vi "test-discretization-13.vi"(8 "error in (no error)":errorcluster) -> (0 "error out":errorcluster, 3 "All Tests Passed":bool)   [LabVIEW 2019]
uses:
  <vilib>/Analysis/Matrix/Datatypes/RealMatrix.ctl
  <vilib>/Analysis/_algsub.llb/Matrix Norm Type.ctl
  <vilib>/Analysis/_algsub.llb/Real Matrix Norm.vi
  <vilib>/Rock Robotics/WPI/ThirdParty/JAS_Junk/TrajLib/MatBuilder_Create.vi
  <vilib>/Rock Robotics/WPI/ThirdParty/JAS_Junk/TrajLib/MatrixHelper_CoerceSize.vi
  <vilib>/Rock Robotics/WPI/ThirdParty/JAS_Junk/TrajLib/Matrix_Transpose.vi
  <vilib>/Rock Robotics/WPI/ThirdParty/JAS_Junk/TrajLib/Matrix_AssignBlock.vi
  <vilib>/Rock Robotics/WPI/ThirdParty/JAS_Junk/TrajLib/Matrix_Exp.vi
  <vilib>/Rock Robotics/WPI/ThirdParty/JAS_Junk/TrajLib/Matrix_Block.vi
  <vilib>/Analysis/baseanly.llb/A x B.vi
  <vilib>/Analysis/baseanly.llb/Real A x B.vi
  <vilib>/Analysis/7linalg.llb/Transpose Matrix.vi
  <vilib>/Analysis/7linalg.llb/Real Transpose Matrix.vi
  <vilib>/Rock Robotics/WPI/ThirdParty/JAS_Junk/TrajLib/Discretization_DiscretizeA.vi
  <vilib>/Analysis/7linalg.llb/Matrix Exp.vi
  <vilib>/Analysis/7linalg.llb/Real Matrix Exp.vi
  <vilib>/Analysis/Matrix/Numeric/Add/Add.vi
  <vilib>/Analysis/Matrix/Numeric/Add/Add - RM,RM.vi
  <vilib>/Analysis/Matrix/Numeric/Multiply/Multiply.vi
  <vilib>/Analysis/Matrix/Numeric/Multiply/Multiply - RM,R.vi
  <vilib>/Analysis/Matrix/Numeric/Subtract/Subtract - RM,RM.vi
  <vilib>/Rock Robotics/WPI/ThirdParty/JAS_Junk/TrajLib/Trajectory_Library.lvlib
  <vilib>/Analysis/Matrix/NI_Matrix.lvlib
  <vilib>/Analysis/NI_AALPro.lvlib
panel:
  out "DiscQ Taylor":T1
  out "DiscA Taylor":T1
  out "DiscA":T1
  out "int DiscQ":T1
  out "ApproxEquals":bool
  in  "Cluster":cluster{"ContQ":T1, "ContA":T1}
  out "DiscQ":T1
  out "norm":dbl format="%.4f"
  out "int discq":bool
  out "Norm error":i32
  out "discAq":bool
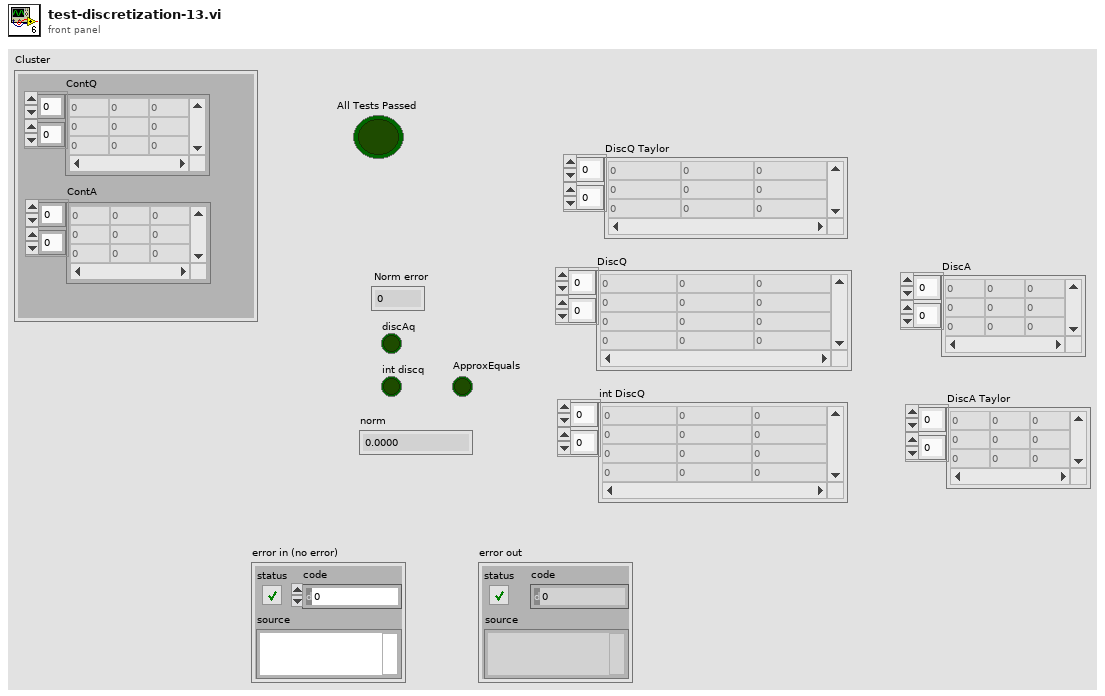
[diagram p1: front panel]
types:
  T1 = typedef "NI_Matrix.lvlib/RealMatrix.ctl" = dbl[][]
  T2 = typedef "NI_AALPro.lvlib/Matrix Norm Type.ctl" = i32
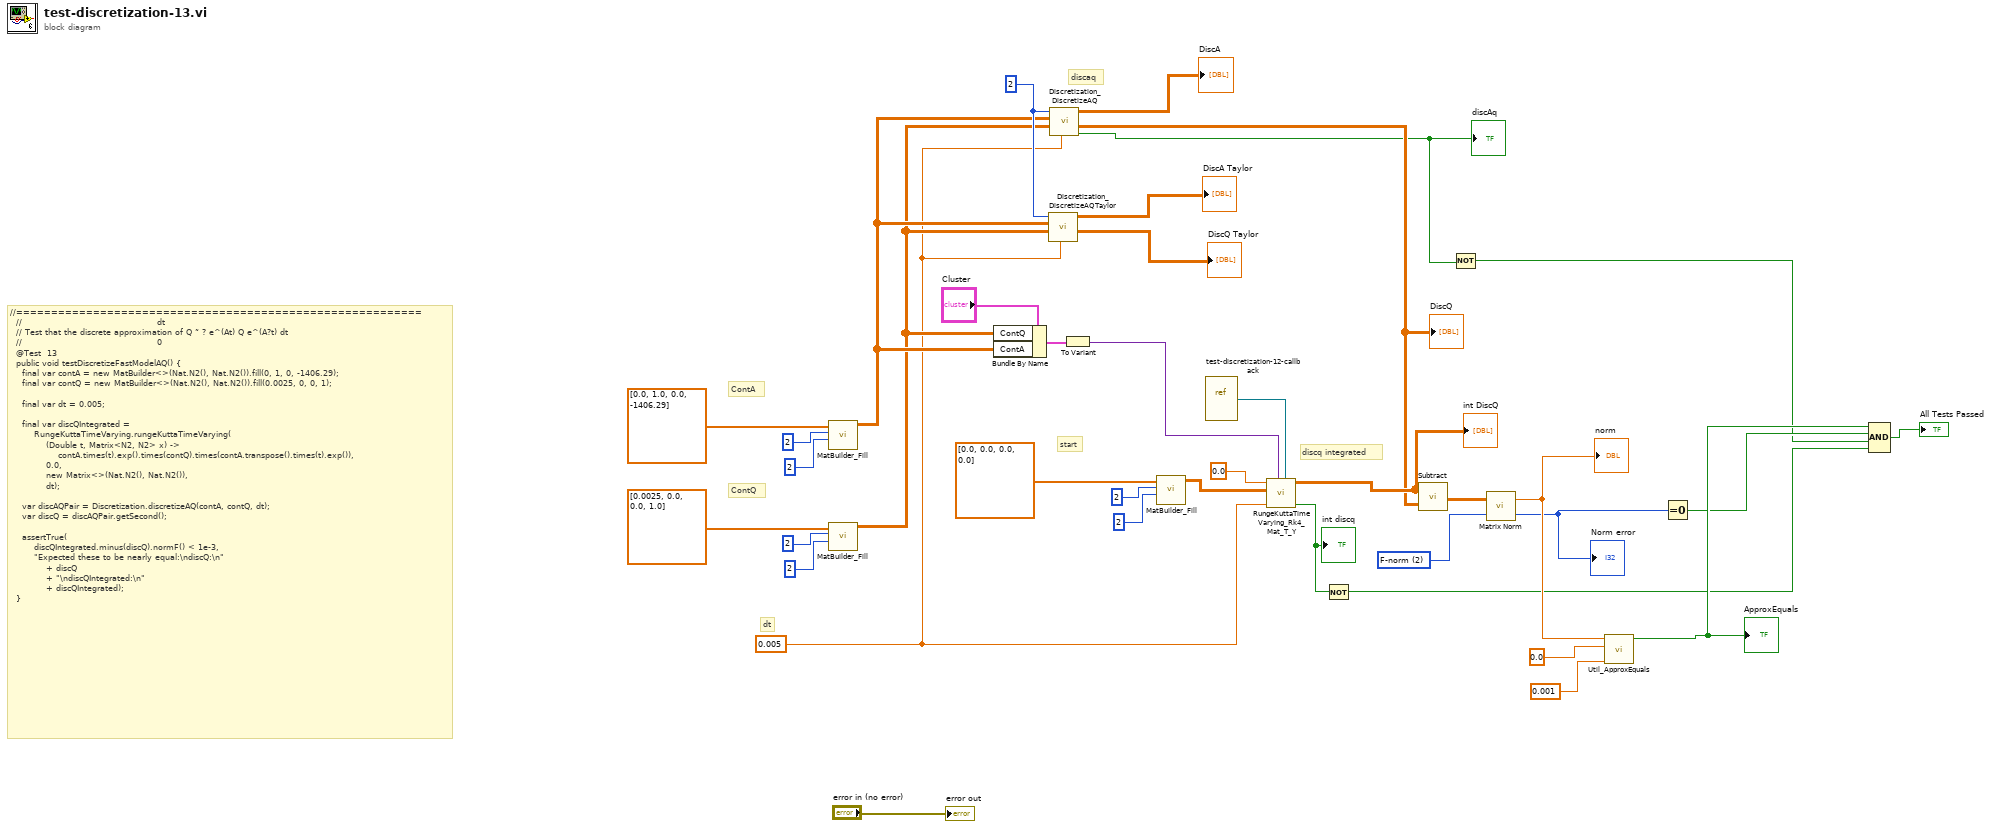
[diagram p0: block diagram]
diagram:
  w6 = 0.005
  w24 = T2 2 items=["2-norm", "1-norm", "F-norm", "Inf-norm"] ("norm type")
  w9 = 2 ("States")
  # "dt"
  # "//==========================================================\n  //                                             dt\n  // Test that the discrete approximation of Q ˜ ? e^(At) Q e^(A?t) dt\n  //                                             0\n  @Test  13\n  public void testDiscretizeFastModelAQ() {\n    final var contA = new MatBuilder<>(Nat.N2(), Nat.N2()).fill(0, 1, 0, -1406.29);\n    final var contQ = new MatBuilder<>(Nat.N2(), Nat.N2()).fill(0.0025, 0, 0, 1);\n\n    final var dt = 0.005;\n\n    final var discQIntegrated =\n        RungeKuttaTimeVarying.rungeKuttaTimeVarying(\n            (Double t, Matrix<N2, N2> x) ->\n                contA.times(t).exp().times(contQ).times(contA.transpose().times(t).exp()),\n            0.0,\n            new Matrix<>(Nat.N2(), Nat.N2()),\n            dt);\n\n    var discAQPair = Discretization.discretizeAQ(contA, contQ, dt);\n    var discQ = discAQPair.getSecond();\n\n    assertTrue(\n        discQIntegrated.minus(discQ).normF() < 1e-3,\n        \"Expected these to be nearly equal:\\ndiscQ:\\n\"\n            + discQ\n            + \"\\ndiscQIntegrated:\\n\"\n            + discQIntegrated);\n  }"
  # "discaq"
  # "discq integrated"
  # "start"
  # "ContQ"
  # "ContA"
  n1 = call <vilib>:"MatBuilder_Fill.vi"("Columns"=2, "Rows"=2, "Value List"=dbl[] [0.0, 1.0, 0.0, -1406.29]) -> ("output matrix"=w8:T1)  [unwired: 8 in]
  n2 = call <vilib>:"MatBuilder_Fill.vi"("Columns"=2, "Rows"=2, "Value List"=dbl[] [0.0025, 0.0, 0.0, 1.0]) -> ("output matrix"=w7:T1)  [unwired: 8 in]
  n3 = Bundle By Name(cluster="Cluster", "ContQ"=w7, "ContA"=w8) -> (w21:cluster{"ContQ":T1, "ContA":T1})
  n4 = call <vilib>:"Discretization_DiscretizeAQTaylor.vi"("dT_Seconds"=w6, "ContQ"=w7, "ContA"=w8, "States"=w9) -> ("DiscQ"=→"DiscQ Taylor":T1, "DiscA"=→"DiscA Taylor":T1)  [unwired: 5 in, 1 out]
  n5 = call <vilib>:"Discretization_DiscretizeAQ.vi"("dT_Seconds"=w6, "ContQ"=w7, "ContA"=w8, "States"=w9) -> ("Error"=w4:bool, "DiscQ"=w5:T1, "DiscA"=→"DiscA":T1)  [unwired: 5 in]
  "discAq" <- w4
  "DiscQ" <- w5
  n6 = To Variant(anything=w21) -> (Variant=w20:variant)
  n7 = call <vilib>:"MatBuilder_Fill.vi"("Columns"=2, "Rows"=2, "Value List"=dbl[] [0.0, 0.0, 0.0, 0.0]) -> ("output matrix"=w26:T1)  [unwired: 8 in]
  n8 = vi-ref "test-discretization-12-callback.vi"() -> (w31:refnum<vi>)
  n9 = call <vilib>:"RungeKuttaTimeVarying_Rk4_Mat_T_Y.vi"("Func_T_Y_Extra"=w31, "PassedData"=w20, "dT_Seconds"=w6, "Y"=w26, "T"=0.0) -> ("Error"=w12:bool, "OUTPUT"=w25:T1)  [unwired: 5 in]
  "int discq" <- w12
  "int DiscQ" <- w25
  n10 = Not(x=w12) -> (.not. x?=w11:bool)
  n11 = call-poly <vilib>:"Subtract.vi"("Real Matrix B"=w5, "Real Matrix A"=w25) -> ("A - B"=w23:T1)
  n12 = Not(x=w4) -> (.not. x?=w13:bool)
  n13 = call-poly <vilib>:"Matrix Norm.vi"("norm type"=w24, "Input Matrix"=w23) -> ("error"=w15:i32, "norm"=w19:dbl)
  "Norm error" <- w15
  "norm" <- w19
  n14 = call <vilib>:"Util_ApproxEquals.vi"("Tolerance"=0.001, "Value 2"=0.0, "Value 1"=w19) -> ("ApproxEquals"=w16:bool)  [unwired: 8 in]
  "ApproxEquals" <- w16
  n15 = Equal To 0?(x=w15) -> (x = 0?=w14:bool)
  n16 = Compound Arithmetic op=AND(w16, w14, w13, w11) -> (→"All Tests Passed":bool)
  "error out" <- "error in (no error)"
